vi "Get Tx Generic Payload List.vi"(8 "error in":errorcluster, 11 "custom device ref in":T3 format="%.0x") -> (0 "error out":errorcluster, 2 "Raw Frame List":T2[](array[typedef]) {"Data" format="%.0x"; "HeaderInfo"."NetSelect" items=["FDX_TX_FRAME_DLY_A"=0, "FDX_TX_FRAME_DLY_B"=1, "FDX_TX_FRAME_BOTH "=3, "FDX_TX_FRAME_ONLY_A"=4, "FDX_TX_FRAME_ONLY_B "=5]; "HeaderInfo"."FrameStartMode" items=["FDX_TX_FRAME_START_IFG", "FDX_TX_FRAME_START_PGWT", "FDX_TX_FRAME_START_TRG"]; "HeaderInfo"."PhysErrorInjection" items=["FDX_TX_FRAME_ERR_OFF"=0, "FDX_TX_FRAME_ERR_CRC"=1, "FDX_TX_FRAME_ERR_ALI"=2, "FDX_TX_FRAME_ERR_PRE"=4, "FDX_TX_FRAME_ERR_PHY"=8]; "HeaderInfo"."SequenceNumberInit" items=["FDX_TX_FRAME_SEQ_INIT_AUTO"=65535]; "HeaderInfo"."SequenceNumberOffset" items=["FDX_TX_FRAME_SEQ_OFFS_AUTO "=65535]; "HeaderInfo"."PayloadGenerationMode" items=["FDX_TX_FRAME_PGM_USER"=0, "FDX_TX_FRAME_PGM_IP_PART"=1, "FDX_TX_FRAME_PGM_IP_FULL"=2, "FDX_TX_FRAME_PGM_IP_PART_TT"=10, "FDX_TX_FRAME_PGM_IP_FULL_TT"=20]; "HeaderInfo"."PayloadBufferMode" items=["FDX_TX_FRAME_PBM_STD", "FDX_TX_FRAME_PBM_MAC", "FDX_TX_FRAME_PBM_UDP"]}, 3 "custom device ref out":T3 format="%.0x", 4 "Found?":bool)   [LabVIEW 2020, in "AIM ARINC 664 Scripting.lvlib"]
uses:
  AIM ARINC 664 Scripting.lvlib
  Constants.vi
  <vilib>/NI VeriStand/Custom Device Tools/Custom Device Utility Library/Custom Device Utility Library.lvlib
  <vilib>/NI VeriStand/Custom Device Tools/Custom Device Utility Library/NI VeriStand - Search for Item by GUID.vi
  <vilib>/NI VeriStand/Custom Device Tools/Custom Device Utility Library/NI VeriStand - Search for All Items by GUID.vi
  <vilib>/NI VeriStand/Custom Device API/Custom Device API.lvlib
  <vilib>/NI VeriStand/Custom Device API/Get Item Property (Variant).vi
  <instrlib>/AIM GmbH/_AIM 664/_controls/queue_header_generic.ctl
  <instrlib>/AIM GmbH/_AIM 664/AIM664LV.lvlib
  <vilib>/NI VeriStand/Custom Device API/Custom Device Item Ref.ctl
  Shared/RawFrame.ctl
panel:
  in  "HeaderInfo":T1 {"NetSelect" items=["FDX_TX_FRAME_DLY_A"=0, "FDX_TX_FRAME_DLY_B"=1, "FDX_TX_FRAME_BOTH "=3, "FDX_TX_FRAME_ONLY_A"=4, "FDX_TX_FRAME_ONLY_B "=5]; "FrameStartMode" items=["FDX_TX_FRAME_START_IFG", "FDX_TX_FRAME_START_PGWT", "FDX_TX_FRAME_START_TRG"]; "PhysErrorInjection" items=["FDX_TX_FRAME_ERR_OFF"=0, "FDX_TX_FRAME_ERR_CRC"=1, "FDX_TX_FRAME_ERR_ALI"=2, "FDX_TX_FRAME_ERR_PRE"=4, "FDX_TX_FRAME_ERR_PHY"=8]; "SequenceNumberInit" items=["FDX_TX_FRAME_SEQ_INIT_AUTO"=65535]; "SequenceNumberOffset" items=["FDX_TX_FRAME_SEQ_OFFS_AUTO "=65535]; "PayloadGenerationMode" items=["FDX_TX_FRAME_PGM_USER"=0, "FDX_TX_FRAME_PGM_IP_PART"=1, "FDX_TX_FRAME_PGM_IP_FULL"=2, "FDX_TX_FRAME_PGM_IP_PART_TT"=10, "FDX_TX_FRAME_PGM_IP_FULL_TT"=20]; "PayloadBufferMode" items=["FDX_TX_FRAME_PBM_STD", "FDX_TX_FRAME_PBM_MAC", "FDX_TX_FRAME_PBM_UDP"]}
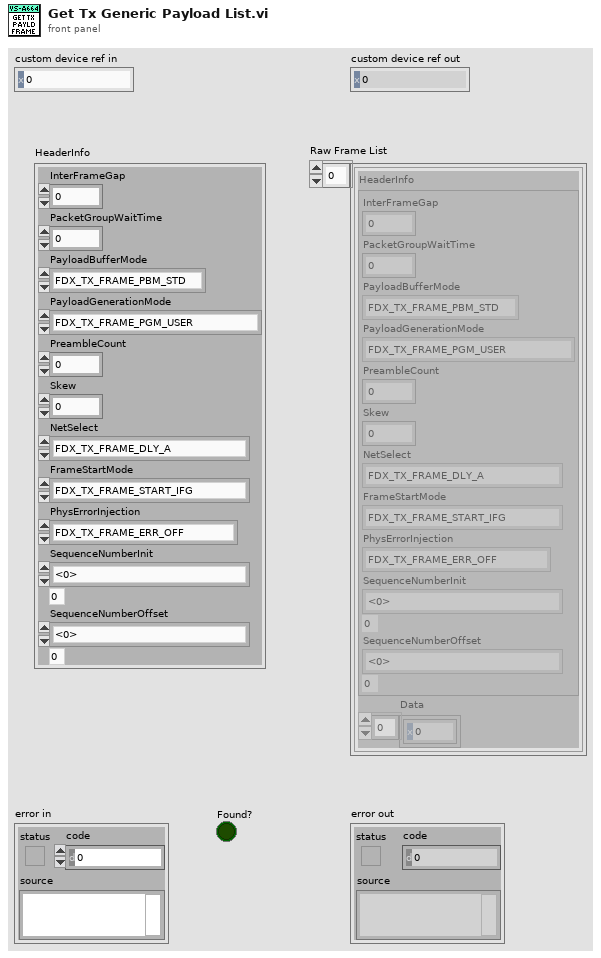
[diagram p1: front panel]
types:
  T1 = typedef "AIM664LV.lvlib/queue_header_generic.ctl" = cluster{"InterFrameGap":u32, "PacketGroupWaitTime":u32, "PayloadBufferMode":u8, "PayloadGenerationMode":u8, "PreambleCount":u8, "Skew":u32, "NetSelect":u8, "FrameStartMode":u8, "PhysErrorInjection":u32, "SequenceNumberInit":u16, "SequenceNumberOffset":u16}
  T2 = typedef "RawFrame.ctl" = cluster{"HeaderInfo":T1, "Data":u8[]}
  T3 = typedef "Custom Device API.lvlib/Custom Device Item Ref.ctl" = u64
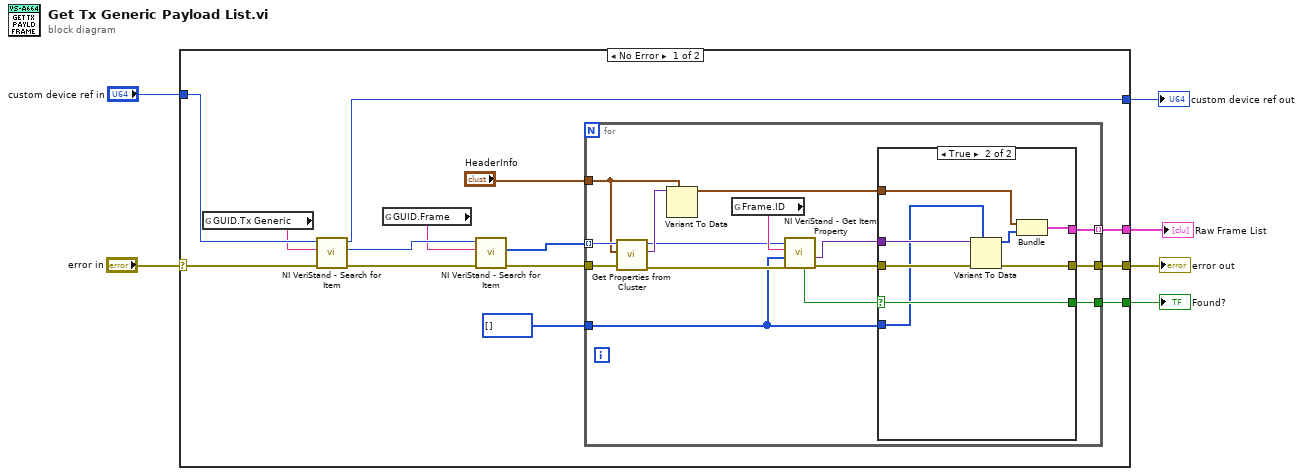
[diagram p0: block diagram]
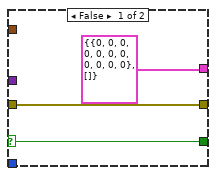
[diagram p2: hidden frame]
diagram:
  n1 = case shown="No Error" "error in" {
    selector: "error in" -> [w19 w48]
    tunnel: "custom device ref in" -> [w20 w47]
    tunnel: [w15 w48] -> w5
    tunnel: [w17 w47] -> w4
    tunnel: [w14 _] -> w1
    tunnel: [w16 _] -> w2
    frame No Error {
      n2 = global read "Constants.vi" "GUID.Tx Generic"() -> (w18:string)
      n3 = call-poly <vilib>:"NI VeriStand - Search for Item.vi"("error in"=w19, "Item GUID"=w18, "Section Ref in"=w20) -> ("error out"=w13:errorcluster, "Item Ref"=w12:T3, "Section Ref out"=w17:T3)  [unwired: 5 in, 1 out]
      n4 = global read "Constants.vi" "GUID.Frame"() -> (w11:string)
      n5 = call-poly <vilib>:"NI VeriStand - Search for Item.vi"("error in"=w13, "Item GUID"=w11, "Section Ref in"=w12) -> ("error out"=w10:errorcluster, "Item Refs"=w9:T3[])  [unwired: 5 in, 2 out]
      n6 = for {
        tunnel: [w33] -> w16
        tunnel: [w31] -> w15
        tunnel: [w30] -> w14 mode=indexing
        tunnel: w10 -> [w29]
        tunnel: w9 -> [w28] mode=indexing
        tunnel: "HeaderInfo" -> [w25]
        tunnel: u8[] [] ("Data") -> [w23]
        n7 = call "Get Properties from Cluster.vi"("error in"=w29, "Variant Cluster"=w25, "custom device ref in"=w28) -> ("error out"=w27:errorcluster, "data"=w26:variant, "custom device ref out"=w21:T3)  [unwired: 5 in, 1 out]
        n8 = Variant To Data(type=w25, Variant=w26) -> (data=w22:T1)  [unwired: 1 in, 1 out]
        n9 = global read "Constants.vi" "Frame.ID"() -> (w35:string)
        n10 = call-poly <vilib>:"NI VeriStand - Get Item Property.vi"("error in (no error)"=w27, "Default Value"=w23, "Property Name"=w35, "Item Ref in"=w21) -> ("error out"=w32:errorcluster, "Value"=w24:variant, "Found?"=w34:bool)  [unwired: 4 in, 1 out]
        n11 = case shown="True" w34 {
          selector: w34 -> [w37 w46]
          tunnel: [w37 w46] -> w33
          tunnel: w32 -> [w38 w45]
          tunnel: [w38 w43] -> w31
          tunnel: [cluster{"HeaderInfo":T1, "Data":u8[]} {"HeaderInfo"={"InterFrameGap"=0, "PacketGroupWaitTime"=0, "PayloadBufferMode"=0, "PayloadGenerationMode"=0, "PreambleCount"=0, "Skew"=0, "NetSelect"=0, "FrameStartMode"=0, "PhysErrorInjection"=0, "SequenceNumberInit"=0, "SequenceNumberOffset"=0}, "Data"=[]} w39] -> w30
          tunnel: w24 -> [_ w44]
          tunnel: w23 -> [_ w42]
          tunnel: w22 -> [_ w41]
          frame False {
          }
          frame True {
            n12 = Variant To Data(error in=w45, type=w42, Variant=w44) -> (data=w40:u8[], error out=w43:errorcluster)
            n13 = Bundle("HeaderInfo"=w41, "Data"=w40) -> (w39:cluster{"HeaderInfo":T1, "Data":u8[]})  [unwired: 1 in]
          }
        }
      }
    }
    frame Error {
    }
  }
  "error out" <- w5
  "custom device ref out" <- w4
  "Found?" <- w2
  "Raw Frame List" <- w1
